vi "Render.IMAQ.TestLauncher.vi"() -> ()   [LabVIEW 2019, in "Render.IMAQ.lvclass"]
uses:
  Render.IMAQ.lvclass
  <vilib>/JKI/JKI SMO/SMO/Typedefs/SMOState --Enum.ctl
  C:/Program Files (x86)/National Instruments/LabVIEW 2019/vi.lib/JKI/JKI SMO/SMO/SMO.lvclass
  <userlib>/LevyLab/Relay Box/Typedefs/Resistor--enum.ctl
  Render.IMAQ.lvclass/Render.IMAQ.ctl
  <vilib>/JKI/JKI SMO/SMO/SMO.lvclass/SMO.ctl
  Typedefs/PrivateEvents--Render.IMAQ.New Background Image.ctl
  <vilib>/JKI/JKI SMO/SMO/Private/ReftoDVR--SMO.vi
  <vilib>/JKI/JKI SMO/SMO/SMO.lvclass
  <userlib>/LevyLab/Relay Box/Relay-Box.lvclass
panel:
  in  "Send Path":bool
  in  "Send Data":bool
  out "Image":T1(plugin-control)
  out "SMO State":T2
  out "error out":errorcluster
  in  "Stop":bool
  # "Basic SMO Test Launcher"
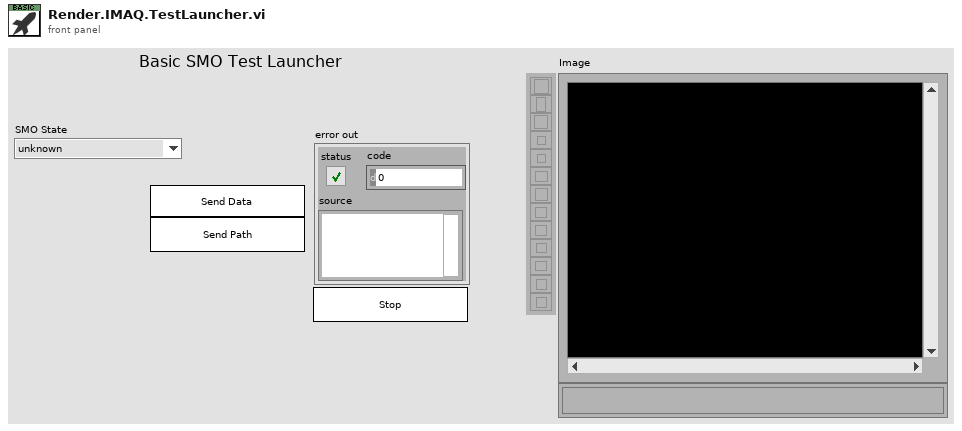
[diagram p1: front panel]
types:
  T1 = typedef "IMAQ Image.ctl" = refnum<image>
  T2 = typedef "SMO.lvclass/SMOState --Enum.ctl" = enum16{"unknown", "Created", "Started", "Stopped"}
  T3 = typedef "Relay-Box.lvclass/Resistor--enum.ctl" = enum16{"open", "discharge tip", "0 ohms", "100k ohm", "10M ohm", "1G ohm"}
  T4 = cluster{"Name":string, "Litho":cluster{"X":dbl, "Y":dbl, "Speed":dbl, "Voltage":dbl}[], "Set Resistance":T3, "Meta":variant}[]
  T5 = typedef "Image Type" = u32
  T6 = typedef "SMO.lvclass/Public Events.ctl" = cluster{"Error":refnum<user-event>, "State":refnum<user-event>, "Reserve State":refnum<user-event>}
  T7 = cluster{"Event Registration Refnum":refnum<event-registration>}
  T8 = typedef "Render.IMAQ.lvclass/PrivateEvents--Render.IMAQ.New Background Image.ctl" = path
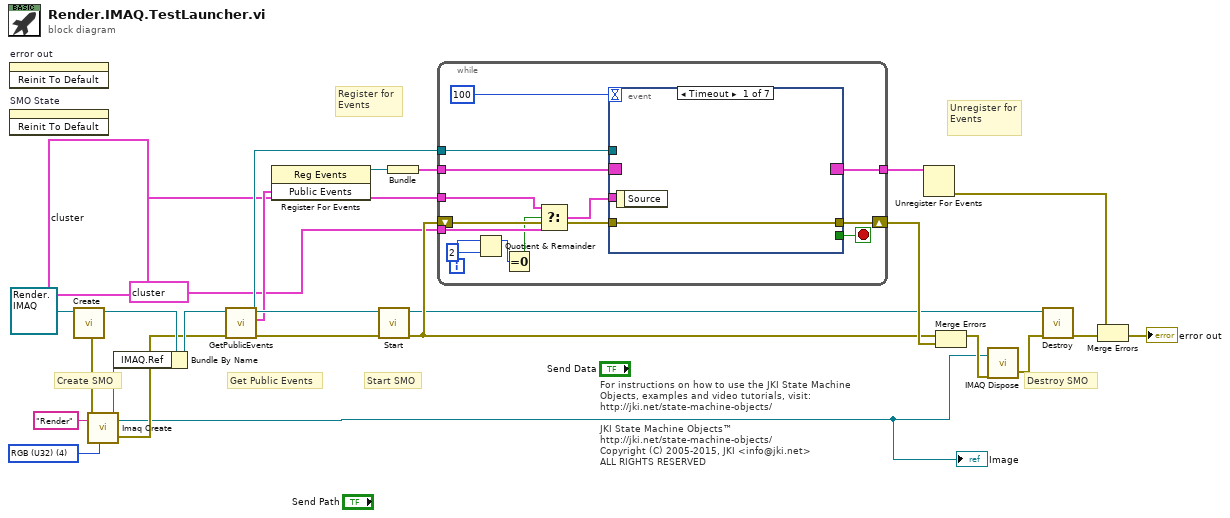
[diagram p0: block diagram]
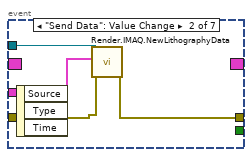
[diagram p2: hidden frame]
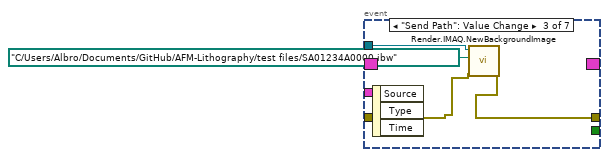
[diagram p3: hidden frame]
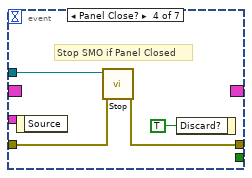
[diagram p4: hidden frame]
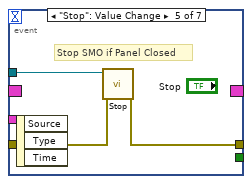
[diagram p5: hidden frame]
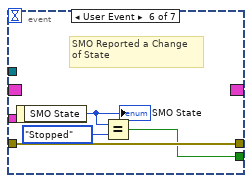
[diagram p6: hidden frame]
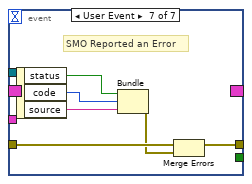
[diagram p7: hidden frame]
diagram:
  w9 = T5 4 items=["Grayscale (U8)", "Grayscale (I16)", "Grayscale (SGL)", "Complex (CSG)", "RGB (U32)", "HSL (U32)", "RGB (U64)", "Grayscale (U16)"] ("Image Type")
  # "For instructions on how to use the JKI State Machine Objects, examples and video tutorials, visit:\nhttp://jki.net/state-machine-objects/\n\nJKI State Machine Objects™\nhttp://jki.net/state-machine-objects/\nCopyright (C) 2005-2015, JKI <info@jki.net>\nALL RIGHTS RESERVED"
  # "Get Public Events"
  # "Start SMO"
  # "Destroy SMO"
  # "Create SMO"
  # "Unregister for Events"
  # "Register for Events"
  n1 = invoke on="error out" class="Clust (strict)" method="Reinit To Default"() -> ()  [unwired: 3 in, 3 out]
  n2 = invoke on="SMO State" class="Enum (strict)" method="Reinit To Default"() -> ()  [unwired: 3 in, 3 out]
  n3 = call <vilib>:"Create.vi"("SMO"=refnum<class "Render.IMAQ.lvclass"> refnum ("SMO.Template.lvclass")) -> ("error out"=w6:errorcluster, "SMO out"=w8:refnum<class "Render.IMAQ.lvclass">)  [unwired: 8 in, 1 out]
  n4 = call "Imaq Create"("Image Name"="Render", "Image Type"=w9, "error in (no error)"=w6) -> ("New Image"=w1:T1, "error out"=w5:errorcluster)  [unwired: 2 in]
  "Image" <- w1
  n5 = Bundle By Name(cluster=w8, "IMAQ.Ref"=w1) -> (w7:refnum<class "Render.IMAQ.lvclass">)
  n6 = call <vilib>:"GetPublicEvents.vi"("error in (no error)"=w5, "SMO"=w7) -> ("error out"=w15:errorcluster, "Public Events"=w13:T6, "SMO out"=w14:refnum<class "Render.IMAQ.lvclass">)  [unwired: 7 in]
  n7 = register-events(w13) -> (reference out=w12:refnum<event-registration>)  [unwired: 2 in, 1 out]
  n8 = call <vilib>:"Start.vi"("error in (no error)"=w15, "SMO"=w14) -> ("error out"=w17:errorcluster, "SMO out"=w16:refnum<class "Render.IMAQ.lvclass">)  [unwired: 8 in]
  n9 = Bundle("Event Registration Refnum"=w12) -> (w23:T7)  [unwired: 1 in]
  n10 = while {
    shift-right: [w37] -> w22
    shift-left: w17 -> [w36]
    tunnel: w23 -> [w35]
    tunnel: [w34] -> w24
    tunnel: w14 -> [w33]
    tunnel: T4 data[2858853B] ("Lithography Data") -> [w25]
    tunnel: T4 data[2858853B] ("Lithography Data") -> [w28]
    i -> [w31]
    stop <- w38 stop-if-true
    n11 = Quotient & Remainder(x=w31, y=2) -> (x-y*floor(x/y)=w29:i32)  [unwired: 1 out]
    n12 = Equal To 0?(x=w29) -> (x = 0?=w27:bool)
    n13 = Select(t=w25, s=w27, f=w28) -> (s? t:f=w26:T4)
    n14 = event shown="[0] Timeout" {
      selector: w35 -> [_ _ _ _ _ _ _]
      dyn-events: [_ _ _ _ _ _ _] -> w34
      timeout: 100 -> [_ _ _ _ _ _ _]
      tunnel: [_ _ _ _ _ w55 _] -> w38
      tunnel: w33 -> [_ w43 w47 w51 w54 _ _]
      tunnel: [w39 w41 w45 w50 w53 w58 w62] -> w37
      tunnel: w36 -> [w39 w40 w46 w49 w52 w58 w60]
      tunnel: w26 -> [_ w42 _ _ _ _ _]
      event Timeout {
        n15 = event-data() -> ()  [unwired: 1 in, 1 out]
      }
      event "Send Data": Value Change {
        n16 = event-data() -> ()  [unwired: 1 in, 3 out]
        n17 = call "Render.IMAQ.NewLithographyData.vi"("error in (no error)"=w40, "NewLithographyData"=w42, "Render.IMAQ"=w43) -> ("error out"=w41:errorcluster)  [unwired: 7 in, 1 out]
      }
      event "Send Path": Value Change {
        n18 = event-data() -> ()  [unwired: 1 in, 3 out]
        n19 = call "Render.IMAQ.NewBackgroundImage.vi"("error in (no error)"=w46, "New Background Image"=T8 path "C:/Users/Albro/Documents/GitHub/AFM-Lithography/test files/SA01234A0000.ibw", "Render.IMAQ"=w47) -> ("error out"=w45:errorcluster)  [unwired: 7 in, 1 out]
      }
      event Panel Close? {
        # "Stop SMO if Panel Closed"
        n20 = event-data() -> ()  [unwired: 1 in, 1 out]
        n21 = call <vilib>:"Stop.vi"("error in (no error)"=w49, "SMO"=w51) -> ("error out"=w50:errorcluster)  [unwired: 8 in, 1 out]
        n22 = event-data("Discard?"=TRUE ("OK")) -> ()  [unwired: 1 in, 1 out]
      }
      event "Stop": Value Change {
        # "Stop SMO if Panel Closed"
        n23 = event-data() -> ()  [unwired: 1 in, 3 out]
        n24 = call <vilib>:"Stop.vi"("error in (no error)"=w52, "SMO"=w54) -> ("error out"=w53:errorcluster)  [unwired: 8 in, 1 out]
      }
      event User Event {
        # "SMO Reported a Change\nof State"
        n25 = event-data() -> ("SMO State"=w57:T2)  [unwired: 1 in]
        "SMO State" <- w57
        n26 = Equal?(x=w57, y=SMOState_--Enum."Stopped") -> (x = y?=w55:bool)
      }
      event User Event {
        # "SMO Reported an Error"
        n27 = event-data() -> ("status"=w61:bool, "code"=w64:i32, "source"=w63:string)  [unwired: 1 in]
        n28 = Bundle("status"=w61, "code"=w64, "source"=w63) -> (w59:errorcluster)  [unwired: 1 in]
        n29 = Merge Errors(w60, w59) -> (w62:errorcluster)
      }
    }
  }
  n30 = Unregister For Events(event registration refnum=w24) -> (error out=w21:errorcluster)  [unwired: 1 in]
  n31 = Merge Errors(w17, w22) -> (w4:errorcluster)
  n32 = call "IMAQ Dispose"("Image"=w1, "error in (no error)"=w4) -> ("error out"=w3:errorcluster)  [unwired: 4 in]
  n33 = call <vilib>:"Destroy.vi"("error in (no error)"=w3, "SMO"=w16) -> ("error out"=w19:errorcluster)  [unwired: 9 in]
  n34 = Merge Errors(w21, w19) -> (→"error out":errorcluster)
